vi "WebView.JSONEditor_Init.vi"(8 "Error In":errorcluster, 10 "WebView2 Control in":refnum<k24>(container), 11 "WebView.JSONEditor in":refnum<class "WebView.JSONEditor.lvclass">) -> (0 "Error Out":errorcluster, 3 "WebView.JSONEditor out":refnum<class "WebView.JSONEditor.lvclass">)   [LabVIEW 2020, in "WebView.JSONEditor.lvclass"]
uses:
  WebView.JSONEditor.lvclass
  WebView.JSONEditor.lvclass/WebView.JSONEditor.ctl
  E:/Git/WebView-Components/Source/Component_class/Component.lvclass
  E:/Git/WebView-Components/Source/WebView.JSONEditor_class/WebView.JSONEditor.lvclass
  private/JSONEditor Events.ctl
  Event Handler.vi
  private/Seleced Node Path Event Data--string.ctl
  private/JSON Updated Event Data--cluster.ctl
  private/Private Events--cluster.ctl
  Component_class/Component.lvclass
  <vilib>/sklein/WebView2/Webview2 Lib/WebView2 Control Object/WebView2 Control.lvclass
  <vilib>/sklein/WebView2/Libs/Microsoft.Web.WebView2.WinForms.dll
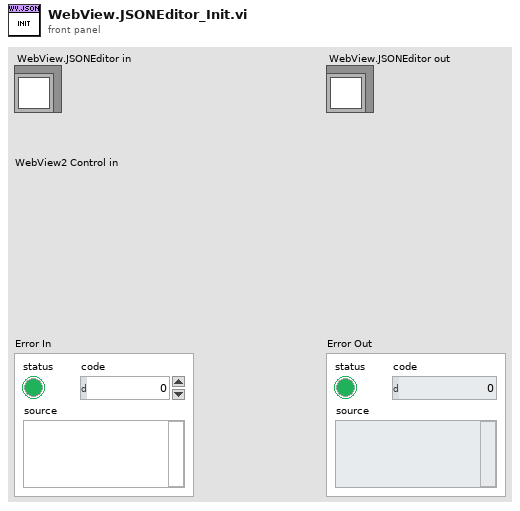
[diagram p1: front panel]
types:
  T1 = typedef "WebView.JSONEditor.lvclass/Private Events--cluster.ctl" = cluster{"Stop Event Handler":refnum<user-event>}
  T2 = typedef "WebView.JSONEditor.lvclass/JSON Updated Event Data--cluster.ctl" = cluster{"JSON":string}
  T3 = typedef "WebView.JSONEditor.lvclass/JSONEditor Events.ctl" = cluster{"JSON Updated":refnum<user-event>, "Selected Node Path":refnum<user-event>}
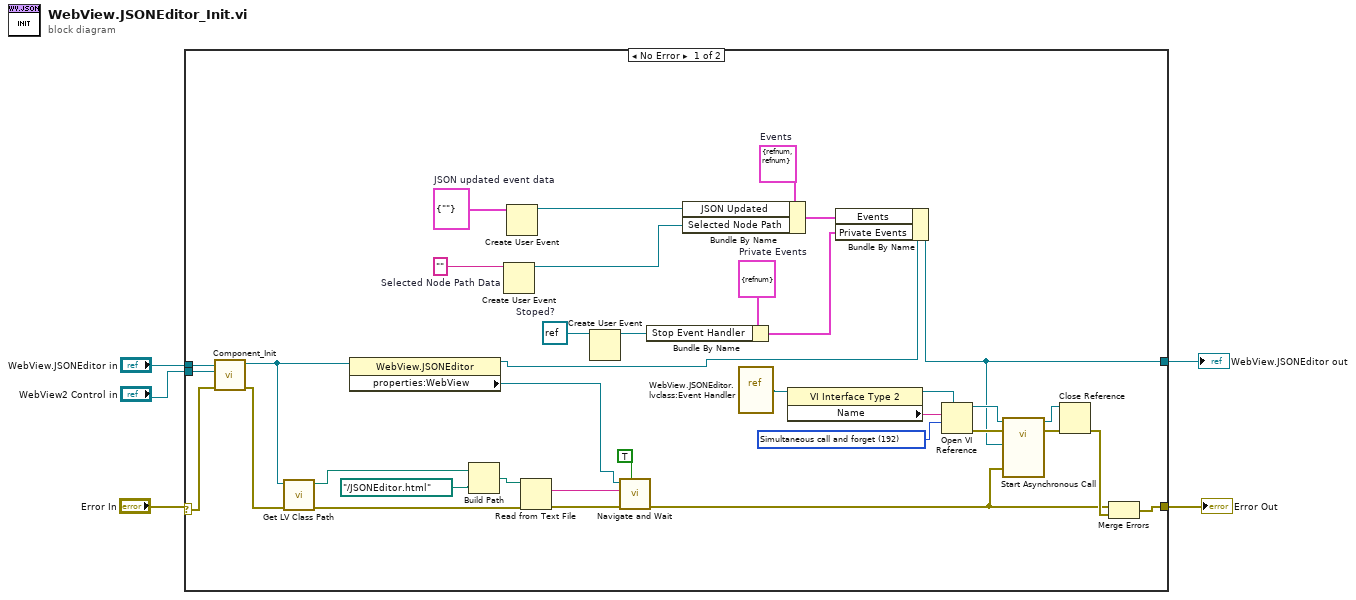
[diagram p0: block diagram]
diagram:
  n1 = case shown="No Error" "Error In" {
    selector: "Error In" -> [w41 w42]
    tunnel: [w18 w43] -> w5
    tunnel: "WebView.JSONEditor in" -> [w40 w43]
    tunnel: [w25 w42] -> w2
    tunnel: "WebView2 Control in" -> [w34 _]
    frame No Error {
      w13 = refnum<notifier> refnum  # Stoped?
      w15 = T1 {"Stop Event Handler"=refnum}  # Private Events
      w17 = T2 {"JSON"=""}  # JSON updated event data
      w22 = T3 {"JSON Updated"=refnum, "Selected Node Path"=refnum}  # Events
      w21 = ""  # Selected Node Path Data
      w26 = 192 items=["Record modifications"=1, "Open templates for editing"=2, "Prompt user to save"=4, "Prepare for reentrant run"=8, "Prompt to find missing subVIs"=16, "Hide loading dialog box"=32, "Enable simultaneous calls"=64, "Prepare to call and forget"=128, "Simultaneous call and forget"=192, "Prepare to call and collect"=256, "Simultaneous call and collect"=320]
      n2 = call "Component_Init.vi"("Error In"=w41, "WebView2"=w34, "object in"=w40) -> ("Error Out"=w39:errorcluster, "object out"=w12:refnum<class "WebView.JSONEditor.lvclass">)  [unwired: 7 in]
      n3 = call <vilib>:"Get LV Class Path.vi"("error in (no error)"=w39, "object"=w12) -> ("error out"=w38:errorcluster, "class path"=w37:path)  [unwired: 8 in]
      n4 = property class="WebView.JSONEditor"(reference=w12) -> (reference out=w10:refnum<class "WebView.JSONEditor.lvclass">, "properties:WebView"=w11:refnum<class "WebView2 Control.lvclass">)  [unwired: 1 in, 1 out]
      n5 = Build Path(base path=w37, name or relative path=path "../JSONEditor.html") -> (appended path=w35:path)
      n6 = Create User Event(user event datatype=w21) -> (user event=w20:refnum<user-event>)  [unwired: 1 in, 1 out]
      n7 = Create User Event(user event datatype=w17) -> (user event=w23:refnum<user-event>)  [unwired: 1 in, 1 out]
      n8 = Read from Text File(file (use dialog)=w35, error in=w38) -> (text=w9:string, error out=w7:errorcluster)  [unwired: 2 in, 2 out]
      n9 = Create User Event(user event datatype=w13) -> (user event=w14:refnum<user-event>)  [unwired: 1 in, 1 out]
      n10 = call <vilib>:"Navigate and Wait.vi"("html Source (URL)"=TRUE, "error in (no error)"=w7, "Source"=w9, "WebView2 Control in"=w11) -> ("error out"=w6:errorcluster)  [unwired: 5 in, 2 out]
      n11 = Bundle By Name(cluster=w15, "Stop Event Handler"=w14) -> (w16:T1)
      n12 = Bundle By Name(cluster=w22, "JSON Updated"=w23, "Selected Node Path"=w20) -> (w19:T3)
      n13 = vi-ref "WebView.JSONEditor.lvclass:Event Handler.vi"() -> (w32:refnum<vi>)
      n14 = property class="VI Interface Type 2"(reference=w32) -> (reference out=w30:refnum<vi>, "Name"=w31:string)  [unwired: 1 in, 1 out]
      n15 = Bundle By Name(cluster=w10, "Events"=w19, "Private Events"=w16) -> (w18:refnum<class "WebView.JSONEditor.lvclass">)
      n16 = Open VI Reference(type specifier VI Refnum (for type only)=w30, vi path=w31, options=w26) -> (vi reference=w33:refnum<vi>, error out=w29:errorcluster)  [unwired: 3 in]
      n17 = call-by-ref "Start Asynchronous Call"(reference=w33, error in=w29, 8:"error in (no error)"=w6, "WebView.JSONEditor in"=w18) -> (reference out=w27:refnum<vi>, error out=w28:errorcluster)  [unwired: 10 in]
      n18 = Close Reference(reference=w27, error in (no error)=w28) -> (error out=w24:errorcluster)
      n19 = Merge Errors(w6, w24) -> (w25:errorcluster)
    }
    frame Error {
    }
  }
  "WebView.JSONEditor out" <- w5
  "Error Out" <- w2
